vi "Convert Angle to Encoder v2.vi"(8 "Floor":dbl, 11 "Angle":dbl) -> (3 "Encoder Units":dbl)   [LabVIEW 2017]
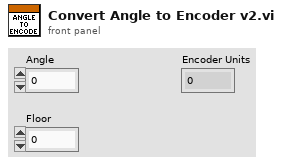
[diagram p1: front panel]
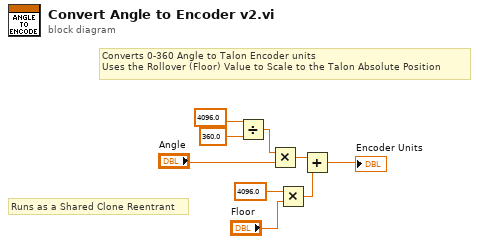
[diagram p0: block diagram]
diagram:
  # "Runs as a Shared Clone Reentrant"
  # "Converts 0-360 Angle to Talon Encoder units\nUses the Rollover (Floor) Value to Scale to the Talon Absolute Position"
  n1 = Divide(x=4096.0, y=360.0) -> (x/y=w9:dbl)
  n2 = Multiply(x=w9, y="Angle") -> (x*y=w6:dbl)
  n3 = Multiply(x=4096.0, y="Floor") -> (x*y=w4:dbl)
  n4 = Add(x=w6, y=w4) -> (x+y=→"Encoder Units":dbl)
